vi "TM_trans (SubVI).vi"(2 "long":dbl format="%#_13g", 3 "lat":dbl format="%#_12g", 4 "ellips":u16(ring) items=["GRS80", "Bessel"]) -> (0 "Y(long)":dbl format="%#_15g", 1 "X(lat)":dbl format="%#_16g")   [LabVIEW 2020]
panel:
  # "NMEA Format"
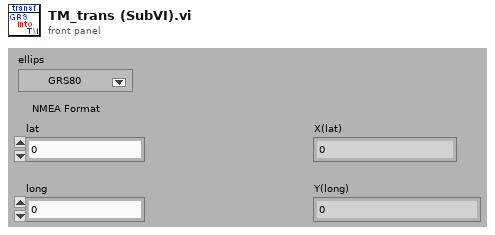
[diagram p1: front panel]
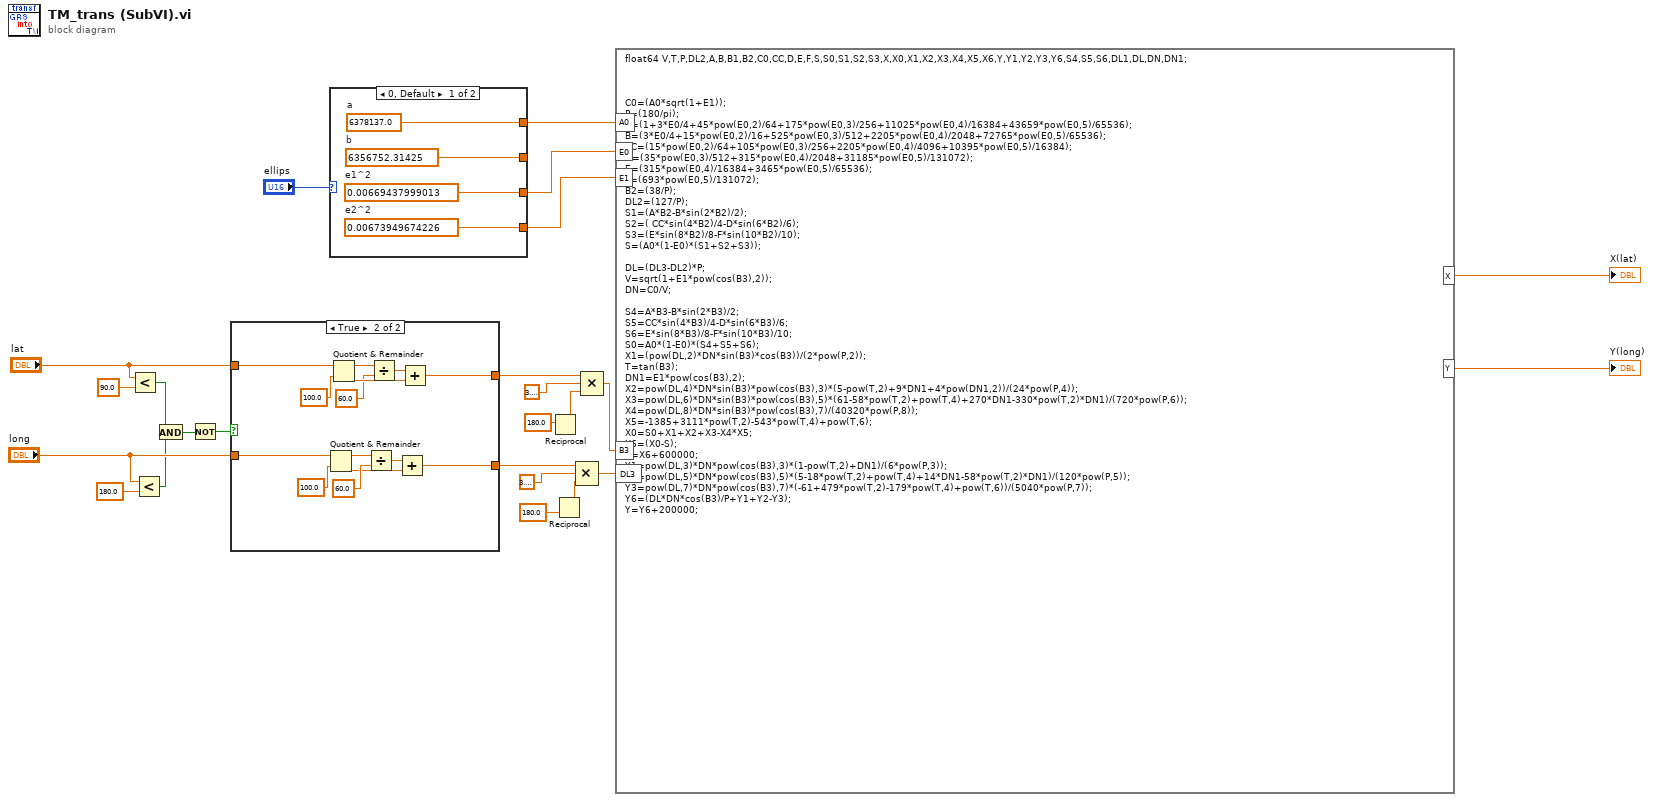
[diagram p0: block diagram]
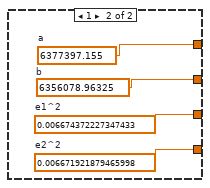
[diagram p3: hidden frame]
diagram:
  n1 = Less?(x="lat", y=90.0) -> (x < y?=w4:bool)
  n2 = Less?(x="long", y=180.0) -> (x < y?=w3:bool)
  n3 = And(x=w4, y=w3) -> (x .and. y?=w2:bool)
  n4 = Not(x=w2) -> (.not. x?=w1:bool)
  n5 = case shown="True" w1 {
    tunnel: "long" -> [w25 w40]
    tunnel: [w25 w39] -> w24
    tunnel: [w26 w33] -> w23
    tunnel: "lat" -> [w26 w32]
    frame False {
    }
    frame True {
      n6 = Quotient & Remainder(x=w40, y=100.0) -> (x-y*floor(x/y)=w36:dbl, floor(x/y)=w35:dbl)
      n7 = Quotient & Remainder(x=w32, y=100.0) -> (x-y*floor(x/y)=w29:dbl, floor(x/y)=w30:dbl)
      n8 = Divide(x=w36, y=60.0) -> (x/y=w38:dbl)
      n9 = Divide(x=w29, y=60.0) -> (x/y=w27:dbl)
      n10 = Add(x=w38, y=w35) -> (x+y=w39:dbl)
      n11 = Add(x=w27, y=w30) -> (x+y=w33:dbl)
    }
  }
  n12 = case shown="0, Default" "ellips" {
    tunnel: [w44 w48] -> w20
    tunnel: [w43 w47] -> _
    tunnel: [w42 w46] -> w21
    tunnel: [w41 w45] -> w22
    frame 0, Default {
      w41 = 0.00673949674226  # e2^2
      w42 = 0.00669437999013  # e1^2
      w43 = 6356752.31425  # b
      w44 = 6378137.0  # a
    }
    frame 1 {
      w45 = 0.006671921879465998  # e2^2
      w46 = 0.006674372227347433  # e1^2
      w47 = 6356078.96325  # b
      w48 = 6377397.155  # a
    }
  }
  n13 = Reciprocal(x=180.0) -> (1/x=w13:dbl)
  n14 = Reciprocal(x=180.0) -> (1/x=w14:dbl)
  n15 = Compound Arithmetic op=MULTIPLY(w24, 3.141592653589793, w14) -> (w18:dbl)
  n16 = Compound Arithmetic op=MULTIPLY(w23, 3.141592653589793, w13) -> (w17:dbl)
  n17 = formula code="float64 V,T,P,DL2,A,B,B1,B2,C0,CC,D,E,F,S,S0,S1,S2,S3,X,X0,X1,X2,X3,X4,X5,X6,Y,Y1,Y2,Y3,Y6,S4,S5,S6,DL1,DL,DN,DN1;\n\n\n\nC0=(A0*sqrt(1+E1)); \nP=(180/pi);                    \nA=(1+3*E0/4+45*pow(E0,2)/64+175*pow(E0,3)/256+11025*pow(E0,4)/16384+43659*pow(E0,5)/65536);     \nB=(3*E0/4+15*pow(E0,2)/16+525*pow(E0,3)/512+2205*pow(E0,4)/2048+72765*pow(E0,5)/65536);\nCC=(15*pow(E0,2)/64+105*pow(E0,3)/256+2205*pow(E0,4)/4096+10395*pow(E0,5)/16384);\nD=(35*pow(E0,3)/512+315*pow(E0,4)/2048+31185*pow(E0,5)/131072);\nE=(315*pow(E0,4)/16384+3465*pow(E0,5)/65536);\nF=(693*pow(E0,5)/131072);\nB2=(38/P);\nDL2=(127/P);\nS1=(A*B2-B*sin(2*B2)/2);\nS2=( CC*sin(4*B2)/4-D*sin(6*B2)/6);\nS3=(E*sin(8*B2)/8-F*sin(10*B2)/10);\nS=(A0*(1-E0)*(S1+S2+S3));\n\nDL=(DL3-DL2)*P;     \nV=sqrt(1+E1*pow(cos(B3),2));\nDN=C0/V;\n\nS4=A*B3-B*sin(2*B3)/2;\nS5=CC*sin(4*B3)/4-D*sin(6*B3)/6;\nS6=E*sin(8*B3)/8-F*sin(10*B3)/10;\nS0=A0*(1-E0)*(S4+S5+S6);\nX1=(pow(DL,2)*DN*sin(B3)*cos(B3))/(2*pow(P,2));\nT=tan(B3);\nDN1=E1*pow(cos(B3),2);\nX2=pow(DL,4)*DN*sin(B3)*pow(cos(B3),3)*(5-pow(T,2)+9*DN1+4*pow(DN1,2))/(24*pow(P,4));\nX3=pow(DL,6)*DN*sin(B3)*pow(cos(B3),5)*(61-58*pow(T,2)+pow(T,4)+270*DN1-330*pow(T,2)*DN1)/(720*pow(P,6));\nX4=pow(DL,8)*DN*sin(B3)*pow(cos(B3),7)/(40320*pow(P,8));\nX5=-1385+3111*pow(T,2)-543*pow(T,4)+pow(T,6);\nX0=S0+X1+X2+X3-X4*X5;\nX6=(X0-S);\nX=X6+600000;\nY1=pow(DL,3)*DN*pow(cos(B3),3)*(1-pow(T,2)+DN1)/(6*pow(P,3));\nY2=pow(DL,5)*DN*pow(cos(B3),5)*(5-18*pow(T,2)+pow(T,4)+14*DN1-58*pow(T,2)*DN1)/(120*pow(P,5));\nY3=pow(DL,7)*DN*pow(cos(B3),7)*(-61+479*pow(T,2)-179*pow(T,4)+pow(T,6))/(5040*pow(P,7));\nY6=(DL*DN*cos(B3)/P+Y1+Y2-Y3);\nY=Y6+200000;"("B3"=w17, "DL3"=w18, "A0"=w20, "E0"=w21, "E1"=w22) -> ("X"=→"X(lat)":dbl, "Y"=→"Y(long)":dbl)
